vi "CarWashTest.vi"(0 "VI Reference In":refnum<vi>, 2 "Label":string, 5 "Wash Option":string, 7 "Car Position":i32=1, 9 "Elapsed Time":dbl=5.0, 11 "error in":errorcluster) -> (4 "VI Reference Out":refnum<vi>, 15 "error out":errorcluster)   [LabVIEW 2016]
uses:
  main/apis/Stimulus/ValueSignal/ValueSignalByPathString.vi
  main/apis/Stimulus/KeyBoardSimulation/ValueSignalLatchBooleanString.vi
  main/apis/Assert/AssertControlValue/True.vi
  main/apis/Assert/AssertControlValue/Equal.vi
  main/apis/Assert/AssertControlValue/AlmostEqual.vi
  <vilib>/addons/_JKI Toolkits/Caraya/classes/Assert/Assert Almost Equal_Float.vi
  main/Drona.lvlib
  main/apis/Stimulus/ValueSignal/ValueSignal.lvlib
  <vilib>/addons/_JKI Toolkits/Caraya/classes/Test/Test.lvclass
  main/apis/Assert/AssertControlValue/AssertControlValue.lvlib
  <vilib>/addons/_JKI Toolkits/Caraya/classes/Assert/Assert.lvclass
  main/apis/Stimulus/KeyBoardSimulation/KeyboardSimulation.lvlib
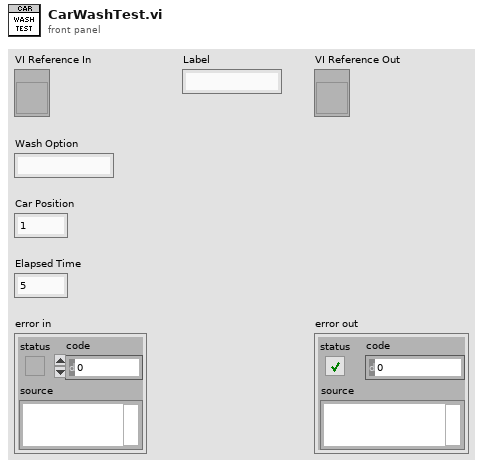
[diagram p1: front panel]
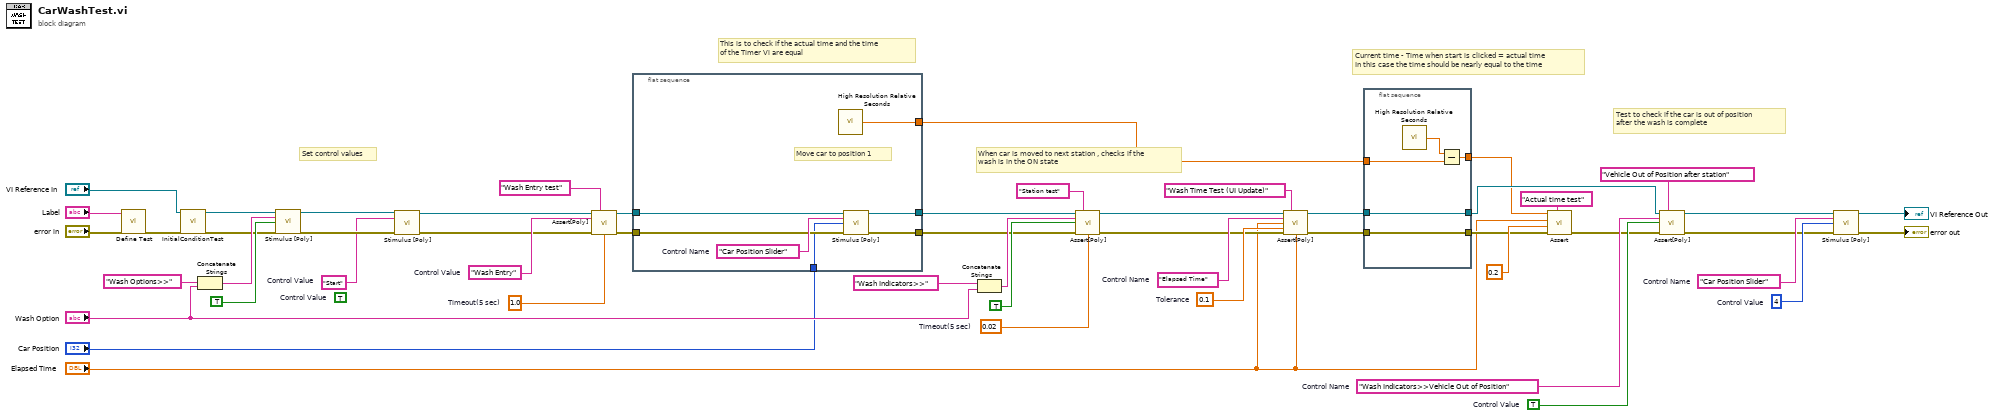
[diagram p0: block diagram]
diagram:
  w24 = "Start"  # Control Value
  (unwired) TRUE  # Control Value
  w36 = 4  # Control Value
  w37 = "Car Position Slider"  # Control Name
  w40 = TRUE  # Control Value
  w47 = 0.02  # Timeout(5 sec)
  w44 = 0.1  # Tolerance
  w45 = "Elapsed Time"  # Control Name
  w41 = "Wash Indicators>>Vehicle Out of Position"  # Control Name
  w51 = 1.0  # Timeout(5 sec)
  w52 = "Wash Entry"  # Control Value
  # "Current time - Time when start is clicked = actual time\nIn this case the time should be nearly equal to the time"
  # "This is to check if the actual time and the time \nof the Timer Vi are equal"
  # "Set control values"
  # "Test to check if the car is out of position \nafter the wash is complete"
  # "When car is moved to next station , checks if the\nwash is in the ON state"
  n1 = call <vilib>:"Define Test.vi"("error in (no error)"="error in", "Label (VI Title)"="Label") -> ("error out"=w14:errorcluster)  [unwired: 9 in]
  n2 = call "InitialConditionTest.vi"("VI Reference In"="VI Reference In", "error in"=w14) -> ("VI Reference Out"=w11:refnum<vi>, "error out"=w13:errorcluster)  [unwired: 12 in]
  n3 = Concatenate Strings("Wash Options>>", "Wash Option") -> (w32:string)
  n4 = call-poly "Stimulus [Poly].vi"("VI Reference In"=w11, "Control Path"=w32, "Value (Signaling)"=TRUE, "error in"=w13) -> ("VI Reference Out"=w27:refnum<vi>, "error out"=w29:errorcluster)  [unwired: 10 in]
  n5 = call-poly "Stimulus [Poly].vi"("VI Reference In"=w27, "Control Path"=w24, "error in"=w29) -> ("VI Reference Out"=w25:refnum<vi>, "error out"=w28:errorcluster)  [unwired: 11 in]
  n6 = call-poly "Assert[Poly].vi"("VI Reference In"=w25, "Label"="Wash Entry test", "Control Path"=w52, "Error In"=w28, "Timeout(5 sec)"=w51) -> ("VI Reference Out"=w49:refnum<vi>, "Error Out"=w50:errorcluster)  [unwired: 9 in]
  n7 = flat-sequence {
    tunnel: w50 -> [w58]
    tunnel: w49 -> [w57]
    tunnel: [w56] -> w38
    tunnel: "Car Position" -> [w55]
    tunnel: [w54] -> w17
    tunnel: [w53] -> w7
    frame #0 {
      w59 = "Car Position Slider"  # Control Name
      # "Move car to position 1"
      n8 = call <vilib>:"High Resolution Relative Seconds.vi"() -> ("relative seconds"=w53:dbl)
      n9 = call-poly "Stimulus [Poly].vi"("VI Reference In"=w57, "Control Path"=w59, "Value (Signaling)"=w55, "error in"=w58) -> ("VI Reference Out"=w56:refnum<vi>, "error out"=w54:errorcluster)  [unwired: 10 in]
    }
  }
  n10 = Concatenate Strings("Wash Indicators>>", "Wash Option") -> (w22:string)
  n11 = call-poly "Assert[Poly].vi"("VI Reference In"=w38, "Label"="Station test", "Control Path"=w22, "Control Value"=TRUE, "Error In"=w17, "Timeout(5 sec)"=w47) -> ("VI Reference Out"=w43:refnum<vi>, "Error Out"=w18:errorcluster)  [unwired: 8 in]
  n12 = call-poly "Assert[Poly].vi"("VI Reference In"=w43, "Label"="Wash Time Test (UI Update)", "Control Path"=w45, "Control Value"="Elapsed Time", "Tolerance"=w44, "Error In"=w18, "Timeout(5 sec)"="Elapsed Time") -> ("VI Reference Out"=w9:refnum<vi>, "Error Out"=w10:errorcluster)  [unwired: 7 in]
  n13 = flat-sequence {
    tunnel: [w64] -> w2
    tunnel: w10 -> [w64]
    tunnel: [w63] -> w8
    tunnel: w9 -> [w63]
    tunnel: w7 -> [w61]
    tunnel: [w60] -> w4
    frame #0 {
      n14 = call <vilib>:"High Resolution Relative Seconds.vi"() -> ("relative seconds"=w62:dbl)
      n15 = Subtract(x=w62, y=w61) -> (x-y=w60:dbl)
    }
  }
  n16 = call-poly <vilib>:"Assert.vi"("Label"="Actual time test", "error in (no error)"=w2, "Tolerance"=0.2, "Y"="Elapsed Time", "X"=w4) -> ("error out"=w3:errorcluster)  [unwired: 6 in]
  n17 = call-poly "Assert[Poly].vi"("VI Reference In"=w8, "Label"="Vehicle Out of Position after station", "Control Path"=w41, "Control Value"=w40, "Error In"=w3) -> ("VI Reference Out"=w35:refnum<vi>, "Error Out"=w34:errorcluster)  [unwired: 9 in]
  n18 = call-poly "Stimulus [Poly].vi"("VI Reference In"=w35, "Control Path"=w37, "Value (Signaling)"=w36, "error in"=w34) -> ("VI Reference Out"=→"VI Reference Out":refnum<vi>, "error out"=→"error out":errorcluster)  [unwired: 10 in]
